vi "图片显示.vi"(1 "图片 in":picture) -> ()   [LabVIEW 2018]
panel:
  out "图片 show":picture
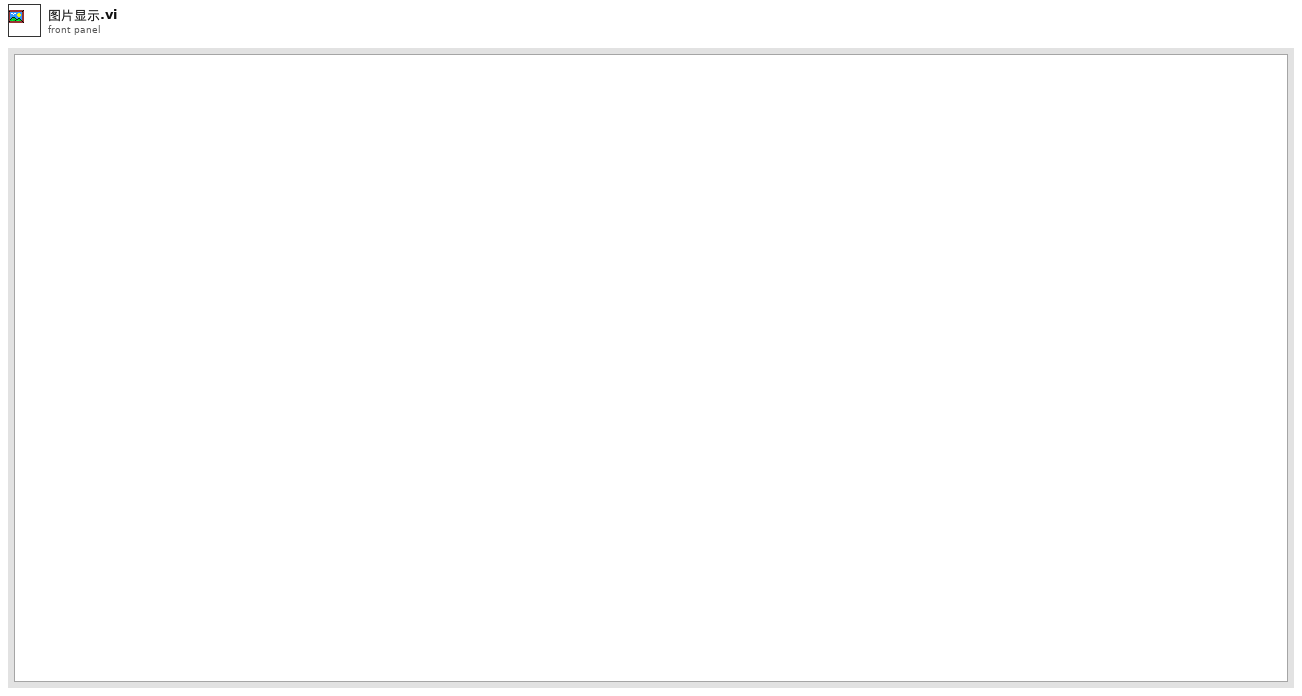
[diagram p1: front panel]
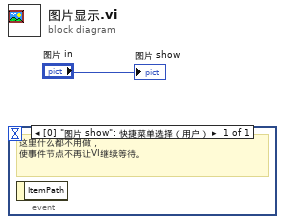
[diagram p0: block diagram]
diagram:
  n1 = event shown="[0] \"图片 show\": 快捷菜单选择（用户）" {
    selector: _ -> [_]
    dyn-events: _ -> [_]
    timeout: _ -> [_]
    event "图片 show": Shortcut Menu Selection (User) {
      # "这里什么都不用做，\n使事件节点不再让VI继续等待。"
      n2 = event-data() -> ()  [unwired: 1 in, 1 out]
    }
  }
  "图片 show" <- "图片 in"
